vi "Write configure scan engine.vi"(8 "error in (no error)":errorcluster, 10 "configure scan engine":bool=TRUE, 11 "Scan Engine configuration1 in":refnum<class "Scan Engine configuration.lvclass">) -> (0 "error out":errorcluster, 3 "Scan Engine configuration1 out":refnum<class "Scan Engine configuration.lvclass">)   [LabVIEW 2013, in "Scan Engine configuration.lvclass"]
uses:
  Scan Engine configuration.lvclass
  Scan Engine configuration.lvclass/Scan Engine configuration.ctl
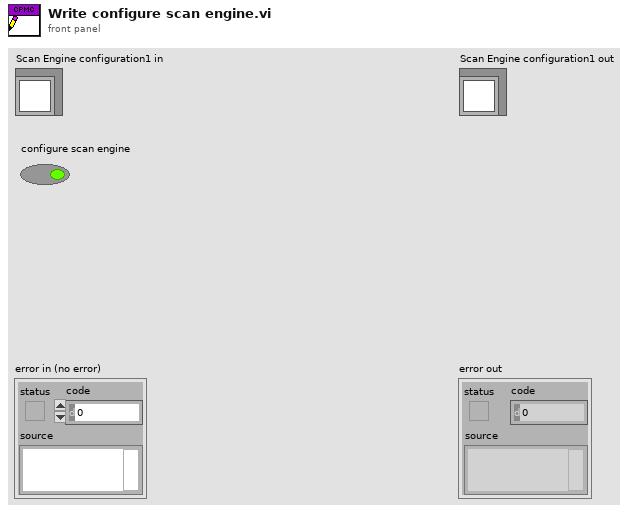
[diagram p1: front panel]
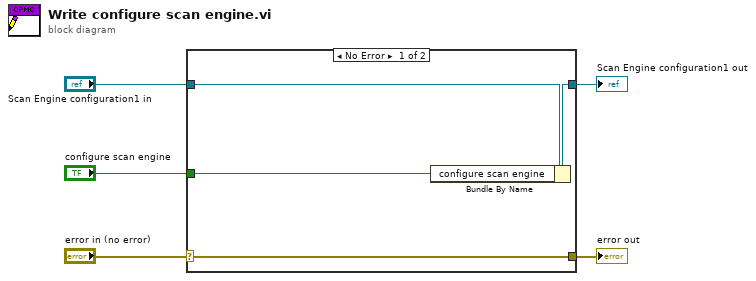
[diagram p0: block diagram]
diagram:
  n1 = case shown="No Error" "error in (no error)" {
    selector: "error in (no error)" -> [w9 w10]
    tunnel: [w9 w10] -> w4
    tunnel: [w7 w11] -> w2
    tunnel: "Scan Engine configuration1 in" -> [w8 w11]
    tunnel: "configure scan engine" -> [w6 _]
    frame No Error {
      n2 = Bundle By Name(cluster=w8, "configure scan engine"=w6) -> (w7:refnum<class "Scan Engine configuration.lvclass">)
    }
    frame Error {
    }
  }
  "error out" <- w4
  "Scan Engine configuration1 out" <- w2
